vi "tm_getdcimgframe.vi"(8 "error in (no error)":errorcluster, 10 "Frame Index":i32=-1, 11 "File Handle in":u32) -> (0 "error out":errorcluster, 1 "Time Sec":dbl, 2 "Data":u16[][](array[numeric]), 3 "File Handle out":u32)   [LabVIEW 2015]
uses:
  tmcamcon.dll
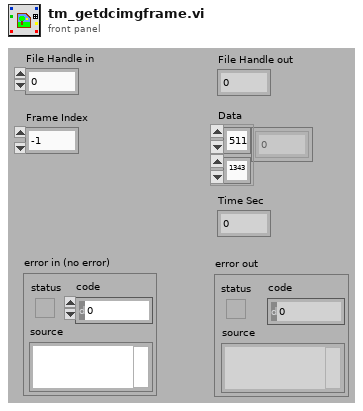
[diagram p1: front panel]
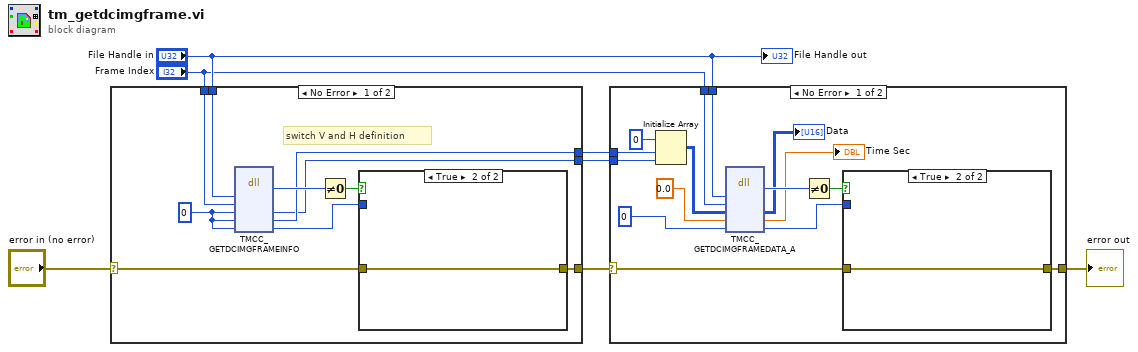
[diagram p0: block diagram]
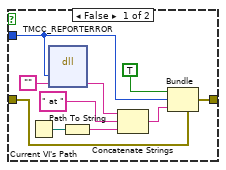
[diagram p2: hidden frame]
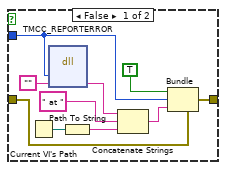
[diagram p4: hidden frame]
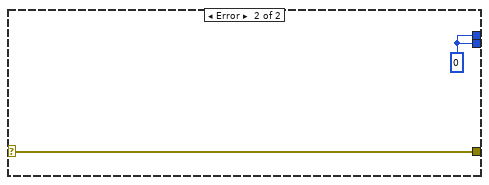
[diagram p5: hidden frame]
diagram:
  n1 = case shown="No Error" "error in (no error)" {
    selector: "error in (no error)" -> [w14 w30]
    tunnel: [w13 w30] -> w6
    tunnel: "File Handle in" -> [w12 _]
    tunnel: [w8 w29] -> w3
    tunnel: [w9 w29] -> w4
    tunnel: "Frame Index" -> [w10 _]
    frame No Error {
      w11 = 0 ("Erval")
      # "switch V and H definition"
      n2 = dll-call lib="tmcamcon.dll" fn="TMCC_GETDCIMGFRAMEINFO"("index"=w12, "frameindex"=w10, "width"=w11, "height"=w11, "Erval"=w11) -> ("return type"=w17:u32, "width"=w8:i32, "height"=w9:i32, "Erval"=w15:i32)  [unwired: 5 in, 2 out]
      n3 = Not Equal To 0?(x=w17) -> (x != 0?=w16:bool)
      n4 = case shown="True" w16 {
        tunnel: w14 -> [w27 w28]
        tunnel: [w26 w28] -> w13
        tunnel: w15 -> [w20 _]
        frame False {
          n5 = Current VI's Path() -> (path=w25:path)
          n6 = dll-call lib="tmcamcon.dll" fn="TMCC_REPORTERROR"("error"=w20, "buf"="") -> ("buf"=w19:string)  [unwired: 5 in, 2 out]
          n7 = Path To String(path=w25) -> (string=w21:string)
          n8 = Concatenate Strings(w19, " at ", w21) -> (w24:string)
          n9 = Bundle(cluster=w27, "status"=TRUE, "code"=w20, "source"=w24) -> (w26:errorcluster)
        }
        frame True {
        }
      }
    }
    frame Error {
      w29 = 0 ("buf")
    }
  }
  n10 = case shown="No Error" w6 {
    selector: w6 -> [w42 w57]
    tunnel: [w41 w57] -> w2
    tunnel: "File Handle in" -> [w40 _]
    tunnel: w4 -> [w38 _]
    tunnel: w3 -> [w37 _]
    tunnel: "Frame Index" -> [w34 _]
    frame No Error {
      n11 = Initialize Array(u16 0 ("buf"), w38, w37) -> (w36:u16[][])
      n12 = dll-call lib="tmcamcon.dll" fn="TMCC_GETDCIMGFRAMEDATA_A"("index"=w40, "frame"=w34, "imgarray"=w36, "timestamp"=0.0 ("Erval"), "Erval"=0) -> ("return type"=w45:u32, "imgarray"=→"Data":u16[][], "timestamp"=→"Time Sec":dbl, "Erval"=w43:i32)  [unwired: 5 in, 2 out]
      n13 = Not Equal To 0?(x=w45) -> (x != 0?=w44:bool)
      n14 = case shown="True" w44 {
        tunnel: w42 -> [w55 w56]
        tunnel: [w54 w56] -> w41
        tunnel: w43 -> [w48 _]
        frame False {
          n15 = Current VI's Path() -> (path=w53:path)
          n16 = dll-call lib="tmcamcon.dll" fn="TMCC_REPORTERROR"("error"=w48, "buf"="") -> ("buf"=w47:string)  [unwired: 5 in, 2 out]
          n17 = Path To String(path=w53) -> (string=w49:string)
          n18 = Concatenate Strings(w47, " at ", w49) -> (w52:string)
          n19 = Bundle(cluster=w55, "status"=TRUE, "code"=w48, "source"=w52) -> (w54:errorcluster)
        }
        frame True {
        }
      }
    }
    frame Error {
    }
  }
  "error out" <- w2
  "File Handle out" <- "File Handle in"
